vi "Get-number-of-clients.vi"(8 "error in (no error)":errorcluster, 10 "Module type":T1, 11 "ModComm in":T2) -> (0 "error out":errorcluster, 2 "# clients":i32, 3 "ModComm out":T2)   [LabVIEW 2013, in "Server.lvlib" / "Server.lvclass"]
uses:
  Server.lvclass
  Object-reference.ctl
  Supported-module-types.ctl
  Server.lvclass/Server.ctl
  Read Clients.vi
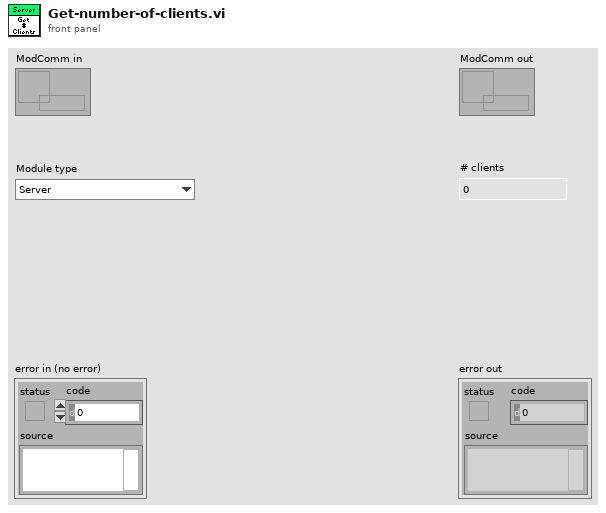
[diagram p1: front panel]
types:
  T1 = typedef "Server.lvlib/Server.lvclass/Supported-module-types.ctl" = enum16{"Server", "All", "BeamControl", "PowderDeposition", "StrategyParser", "CameraVision", "MaterialCharacterization", "StatusMonitor", "SLMSimulation", "LaserCharacterization"}
  T2 = typedef "Server.lvlib/Server.lvclass/Object-reference.ctl" = refnum<data-value>
  T3 = typedef "Module-communication.lvlib/Server.lvclass/Supported-module-types.ctl" = enum16{"Server", "All", "BeamControl", "PowderDeposition", "StrategyParser", "CameraVision", "MaterialCharacterization", "StatusMonitor", "SLMSimulation", "LaserCharacterization"}
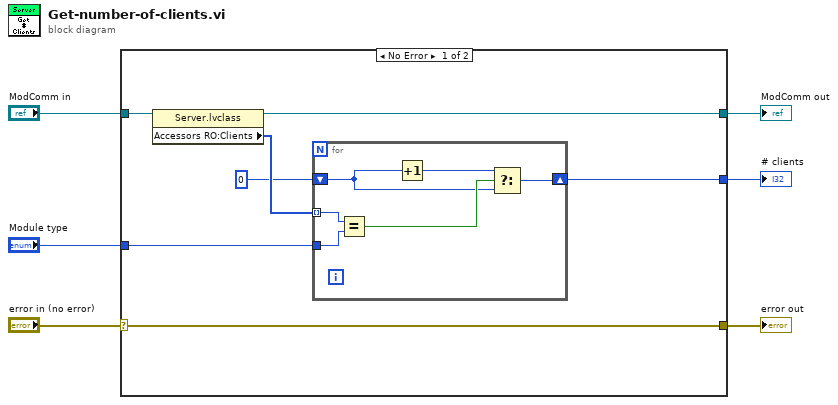
[diagram p0: block diagram]
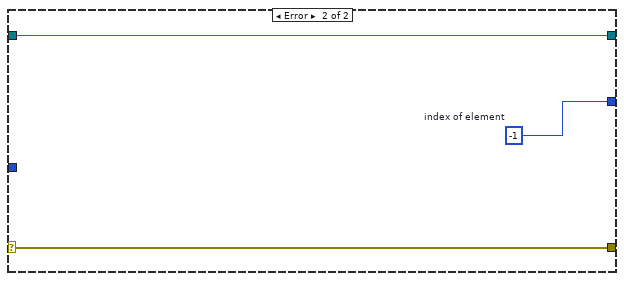
[diagram p2: hidden frame]
diagram:
  n1 = case shown="No Error" "error in (no error)" {
    selector: "error in (no error)" -> [w13 w22]
    tunnel: [w13 w22] -> w5
    tunnel: [w11 w21] -> w3
    tunnel: "ModComm in" -> [w12 w21]
    tunnel: "Module type" -> [w9 _]
    tunnel: [w7 w20] -> w1
    frame No Error {
      n2 = property class="Server.lvclass"(reference=w12) -> (reference out=w11:T2, "Accessors RO:Clients"=w10:T3[])  [unwired: 1 in, 1 out]
      n3 = for {
        tunnel: w10 -> [w16] mode=indexing
        tunnel: w9 -> [w19]
        shift-right: [w18] -> w7
        shift-left: 0 -> [w15]
        n4 = Equal?(x=w16, y=w19) -> (x = y?=w17:bool)
        n5 = Increment(x=w15) -> (x+1=w14:i32)
        n6 = Select(t=w14, s=w17, f=w15) -> (s? t:f=w18:i32)
      }
    }
    frame Error {
      w20 = -1  # index of element
    }
  }
  "error out" <- w5
  "ModComm out" <- w3
  "# clients" <- w1
